vi "Read Invalid Event.vi"(8 "error in (no error)":errorcluster, 11 "OnChangeNotifier_Boolean in":refnum<class "OnChangeNotifier_CDBL.lvclass">) -> (0 "error out":errorcluster, 2 "Invalid Event":bool, 3 "OnChangeNotifier_Boolean out":refnum<class "OnChangeNotifier_CDBL.lvclass">)   [LabVIEW 2021, in "OnChangeNotifier_CDBL.lvclass"]
uses:
  OnChangeNotifier_CDBL.lvclass
  OnChangeNotifier_CDBL.lvclass/OnChangeNotifier_CDBL.ctl
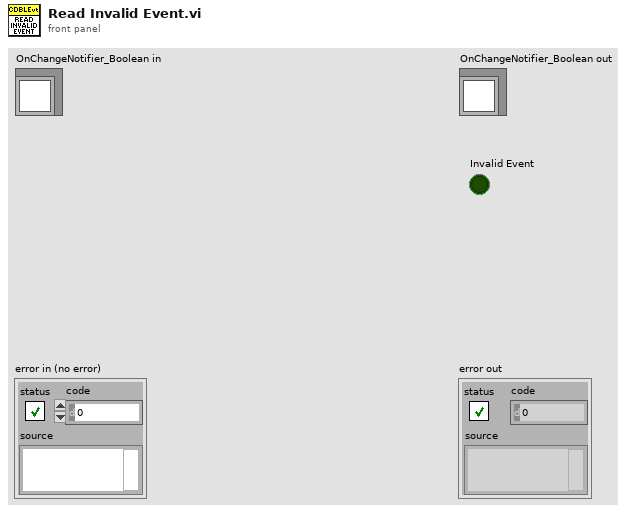
[diagram p1: front panel]
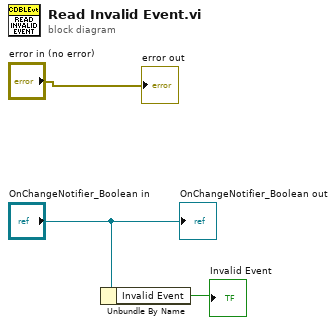
[diagram p0: block diagram]
diagram:
  n1 = Unbundle By Name("OnChangeNotifier_Boolean in") -> ("Invalid Event"=→"Invalid Event":bool)
  "error out" <- "error in (no error)"
  "OnChangeNotifier_Boolean out" <- "OnChangeNotifier_Boolean in"
